vi "Query Arb Waveform Capabilities 64 [ARB64] Core.vi"(8 "error in (no error)":errorcluster, 11 "CS++Fgen in":refnum<class "CS++Fgen.lvclass">) -> (0 "error out":errorcluster, 1 "waveform quantum":i32, 2 "max number of waveforms":i32, 3 "CS++Fgen out":refnum<class "CS++Fgen.lvclass">, 4 "max waveform size":i64, 6 "min waveform size":i64)   [LabVIEW 2013, in "CS++Fgen.lvlib" / "CS++Fgen.lvclass"]
doc: "This VI returns the properties of the function generator that are related to creating arbitrary waveforms. These properties are the maximum number of waveforms, waveform quantum, minimum waveform size, and maximum waveform size.\n\nThis VI is a 64-bit version of IviFgen Query Arb Waveform Capabilities [ARB] VI.\n\nNote:\n\n(1) This VI is part of the IviFgenArbWfmSize64 [ARB64] extension group."
uses:
  CS++Fgen.lvclass
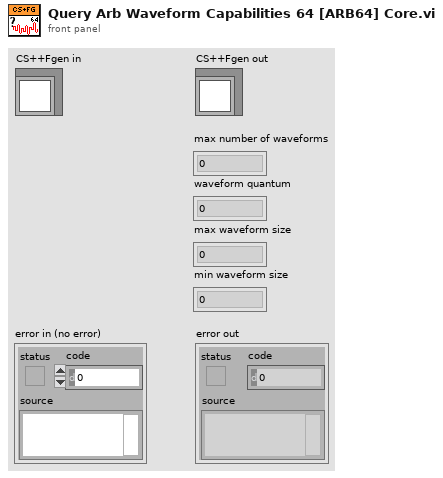
[diagram p1: front panel]
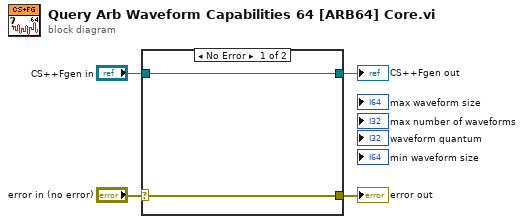
[diagram p0: block diagram]
diagram:
  n1 = case shown="No Error" "error in (no error)" {
    selector: "error in (no error)" -> [w5 w8]
    tunnel: [w5 w8] -> w3
    tunnel: [w6 w7] -> w1
    tunnel: "CS++Fgen in" -> [w6 w7]
    frame No Error {
    }
    frame Error {
    }
  }
  "error out" <- w3
  "CS++Fgen out" <- w1
